vi "File Viewer v2.vi"() -> ()   [LabVIEW 2019]
uses:
  <vilib>/Utility/file.llb/Read Delimited Spreadsheet (I64).vi
panel:
  in  "Stop":bool
  in  "Tab Control":T1(tab)
  out "Raw Image From Camera":i32[][](graph)
  in  "file path for picture":path
  out "Expected position on spectrometer (pixels):":dbl
  in  "Grating:":u16(ring) items=["Shimadzu 30-006  "]
  in  "Laser:":u16(ring) items=["800nm  "]
  in  "Harmonic":dbl min=10.0 max=40.0
  out "l (nm)":dbl
  out "E (J)":dbl
  out "E (eV)":dbl
  out "Nearest Harmonic of 800nm":dbl
  out "Vertical Binned Waveform Graph":i64[](graph)
  out "Cursor Position (pixels)":dbl
  out "Distance to nearest harmonic of 800nm (pixels)":dbl
  in  "Caibration Date":u16(ring) items=["first calibration - 7/31", "7/31-current"]
  out "Wavelength Graph":cluster{"lamda (m)":dbl, "Numeric":i64}[](graph)
  out "Energy Graph (eV)":cluster{"lamda (m)":dbl, "Numeric":i64}[](graph)
  out "Harmonics Graph":cluster{"lamda (m)":dbl, "Numeric":i64}[](graph)
  in  "Pump/Probe Run Folder:":path
  out "XUV":dbl[][](graph)=[[0.0010313840536425023, 0.0010313840536425023, 0.0010274759814052766, 0.0010401531177745159, 0.00104452387932524, 0.0010522711712232782, 0.001047206375702307, 0.0010453914217880493, 0.0010393489196820073, 0.0010272942106035452, 0.0010408196107141979, 0.0010468510964080136, 0.001062026204249532, 0.001106433361933133, 0.001154520001300267, 0.0011934960677563772, 0.001214033414248973, 0.0012241024150236718, 0.0012391453259184763, 0.0012555680424446059, 0.0012925281054633312, 0.001352528994653044, 0.0014089853532089937, 0.0014660421062312687, 0.0015363130457188075, 0.0015691474623588406, 0.0016108363203256395, 0.0016140062929437132, 0.0015863330654316305, 0.001566139981821102, 0.0015480455247396548, 0.0015630250912641588, 0.0016089194645982896, 0.0016388896140595243, 0.0016752961023638853, 0.001688323009821305, 0.0016919033437948032, 0.0017147706614732288, 0.0017464097973867246, 0.001779717919752482, 0.001837171263614898, 0.00188523587015758, 0.001909243386501412, 0.0019293676175355272, 0.0019505631946586353, 0.0019533283141273984, 0.001977616748982997, 0.0019911972311547808, 0.002017708227177005, 0.002053718124641225, 0.0020883013967221585, 0.002112669700566397, 0.0021315656016372966, 0.0021208218456137463, 0.002105299720787104, 0.002099830072116822, 0.0021012126318512036, 0.0020908214010188896, 0.002095054457416787, 0.002100080695494967, 0.0021084586769929523, 0.0020993728910094368, 0.002104955457905037, 0.0020792872174181134, 0.0020928346503532183, 0.0020942117018814864, 0.002102964241395161, 0.0021093372358679877, 0.002121036665652156, 0.002136567052787968, 0.002154127213876447, 0.002169360157882152, 0.0021869395976920275, 0.0021825908689657556, 0.002171045668952753, 0.0021674267775364637, 0.0021489908116760054, 0.002157660728097984, 0.002145658346977596, 0.002135917084466625, 0.00209696855904108, 0.0020850653256307278, 0.0020535996982097935, 0.002049595232365589, 0.0020524236962046524, 0.0020767176392663643, 0.002111884781195284, 0.002137809153266466, 0.0021668842192343256, 0.00216397037820051, 0.0021656008072099796, 0.0021352698702483386, 0.0021013916485498785, 0.0020823029602650214, 0.0020479290000163844, 0.0020333460243320213, 0.0020002169186649392, 0.0019659586307446764, 0.0019358700548520106, 0.0019274369912928948, 0.0019173046461478957, 0.001900014387158957, 0.0018599917615413628, 0.001814549061108504, 0.0017608991335671654, 0.0017321325271416374, 0.0017011240808280886, 0.0016809695546603515, 0.0016804848325224012, 0.001677022924980334, 0.0016912533754734602, 0.0016999535870290603, 0.0017145172839920274, 0.001701024933118053, 0.0017087557003977521, 0.0017038864461937952, 0.0017154509249281934, 0.0017378638156022909, 0.001773105318313737, 0.0017971238510697952, 0.001824766783448256, 0.0018273914436611356, 0.0018233456662710829, 0.001811169776658133, 0.001808649772361402, 0.0017980740166243004, 0.0017838545825434003, 0.001763256645783561, 0.0017210445082360198, 0.001701132343137258, 0.0016754062664861471, 0.001664623953019805, 0.0016487024832499652, 0.0016273141189128994, 0.0016010950578146683, 0.0015728930425157306, 0.0015352912734848325, 0.0015149109108664593, 0.001483448037548582, 0.0014523514599372237, 0.0014315579818603703, 0.0014274984339550348, 0.0014181675327994876, 0.0014143999198181453, 0.0014053113797315735, 0.0013993515007172275, 0.001408693418285001, 0.0013985390403155494, 0.001397974449188959, 0.0013917694550025816, 0.0013787315311329358, 0.0013626448151797038, 0.0013449083914956062, 0.0013370509354753064, 0.001325880293477993, 0.0013185543793476045, 0.001294420174263172, 0.00127875483607759, 0.0012659041912157889, 0.0012433398248735822, 0.001228894554342046, 0.0012003400138518715, 0.001183988904005212, 0.0011747543964566436, 0.0011585547622780935, 0.0011605046672421217, 0.0011473565792502146, 0.0011370039058606926, 0.0011340652778993677, 0.0011226770617605876, 0.0011216442731143861, 0.0011107600578349525, 0.0011026409620242816, 0.0010866919512238764, 0.0010731362559796018, 0.001051089661012024, 0.0010301832647098524, 0.001009888279286232, 0.0009965887156262153, 0.0009909235256389188, 0.0009767536654130364, 0.0009747817276245561, 0.0009568910741692924, 0.000949947980363763, 0.000956703795161448, 0.0009593917997446279, 0.0009746082191319944, 0.0009815127554947322, 0.0009862085012061277, 0.0009848589907084247, 0.0009587748806599638, 0.0009397330121270677, 0.0009244532483694009, 0.0009160174307072283, 0.0009138141482619988, 0.0009141501488348964, 0.0009184162544694721, 0.0009130457535092251, 0.000912208506180038, 0.0009004897976744733, 0.0008954966088329721, 0.000888658170943591, 0.000878327530378521, 0.0008779392018475493, 0.0008724833236925496, 0.0008753007711193868, 0.0008733894235981503, 0.0008842763929806406, 0.0008803270091975667, 0.0008834474079606231, 0.0008812331091031674, 0.0008784927765619131, 0.0008838109495640858, 0.0008909550928927427, 0.000899184352825675, 0.0009081654828930417, 0.000914194214483801, 0.0009259542345352136, 0.0009387635678511666, 0.0009425339349355657, 0.0009425063939050002, 0.0009326494590656548, 0.0009267529244216092, 0.0009192645182108854, 0.0009126023429171226, 0.0009054058716303917, 0.0008956756255316468, 0.0008975015958581308, 0.0008902445343041561, 0.0008840973762819658, 0.0008824283898297043, 0.0008799772381093866, 0.000884678492026895, 0.0008933897199947213, 0.0008983829088362226, 0.000893860671617389, 0.0008973749071175302, 0.0009013435696219998, 0.0009055848883290665, 0.0009138995254567515, 0.0009202174378684471, 0.000930589389979365, 0.000922150818214136, 0.0009280666315795773, 0.0009267253833910438, 0.0009243623629685353, 0.0009317653919845064, 0.0009418922289233926, 0.0009494384712983037, 0.0009643051195974898, 0.0009718458537662879, 0.0009862966325039368, 0.0009917001827008621, 0.0009979795376697665, 0.001014038712592433, 0.0010172830459930335, 0.0010330585483008768, 0.0010469640146333317, 0.001060098332109956, 0.0010826544361429932, 0.0011030761103072145, 0.0011350760337211167, 0.0011531154087414334, 0.0011576624328877758, 0.0011768364983673857, 0.0011841624124977737, 0.0011999406689086737, 0.0012165093528967996, 0.0012281895039595726, 0.0012561601746017613, 0.0012707651831105765, 0.001307240523991351, 0.001333627585376031, 0.0013666217399933432, 0.0014024911782016796, 0.0014332324765187446, 0.0014678102403935655, 0.0014988241949132272, 0.0015329365153714935, 0.0015343879276822883, 0.0015720971067323913, 0.0016118636007657278, 0.001651087536496926, 0.0016970920739533186, 0.001745473402347502, 0.0017665615694514051, 0.0018051024876245825, 0.0018256783915599696, 0.0018815618966801597, 0.0018972630382054765, 0.0019475088943689358, 0.001967589059754146, 0.0019944801219981727, 0.0020293085092511383, 0.0020797967264835726, 0.002127649267090901, 0.002177592171918141, 0.002209096356781867, 0.0022576126362258207, 0.0022860239633570555, 0.002367479315357191, 0.00239798651491445, 0.002459918030346795, 0.002492961758819125, 0.0025305745442622493, 0.0025619850896220525, 0.0025918974029190997, 0.0026126908809959533, 0.0026649499864937407, 0.002671884817990101, 0.0027487573425041584, 0.0027664331759210126, 0.0028080311484869457, 0.002835572179052315, 0.002897776350687257, 0.0029281981730497637, 0.0029626547563900967, 0.002993387792397992, 0.0030170785868903222, 0.0030149964849795806, 0.0030319039236436605, 0.0030360240618162396, 0.0030334957952103388, 0.0030378693108641195, 0.003026379192912247, 0.0030242502712495446, 0.0030348563221202682, 0.0030418489897808152, 0.0030719182869520852, 0.0030982750532031434, 0.0030908086798168716, 0.0031010319103627363, 0.0031036813575031253, 0.0030762670156783568, 0.003066933360419753, 0.003042223547796504, 0.0030263378813663996, 0.003004663090311454, 0.0029920548065186284, 0.0029706664421815625, 0.0029578268137319874, 0.0029413352446294445, 0.0029132489016588815, 0.0028961762168114094, 0.002857943758180564, 0.00283680050901553, 0.0028030104186148787, 0.0027938640423641197, 0.0027516161014768444, 0.002719478472910115, 0.0026733913123620267, 0.002627637398283779, 0.0025728335015617514, 0.0025436510255746865, 0.002504355483164018, 0.0024615594757684913, 0.002436053727361903, 0.0024182842544411267, 0.0024007185851465346, 0.0023905779776923655, 0.0023550968680150007, 0.002333292634116398, 0.002292746728918062, 0.0022553735504408563, 0.0022384468330553806, 0.002203128215458351, 0.00217902430550754, 0.002143711196116624, 0.0021122262899742946, 0.0020506142504965077, 0.00203825383597877, 0.0020262487007553258, 0.0020074629638066875, 0.0019932738248594093, 0.0019544327094530695, 0.0019488088310116213, 0.0019049882972790627, 0.0018915620448784454, 0.0018528393559035367, 0.001821197465886984, 0.0017890212798774634, 0.0017354539754278208, 0.0016897689139259869, 0.001663423164087155, 0.0016456371665480398, 0.0016412085688331283, 0.001628644350689207, 0.0016130809143167168, 0.0016073331012377244, 0.001603339651805746, 0.0015941712427305346, 0.001588935692820058, 0.0015824029603699523, 0.00157714813173808, 0.0015643332902160138, 0.0015630746651191763, 0.0015527274999357675, 0.0015555421932595482, 0.0015637163711313498, 0.0015732180266764021, 0.001592557338339404, 0.001584653062567143, 0.0015960522951181493, 0.0016165015103129358, 0.0016268707083207973, 0.0016398039762742945, 0.001641899848700319, 0.0016484215647381982, 0.0016487190078683044, 0.0016555629539637985, 0.0016557612493838694, 0.0016741145921526312, 0.0017004658501975761, 0.0017330110860166727, 0.0017605190673453631, 0.0017664348807108045, 0.0017779084740443371, 0.001790398331405732, 0.0018131775177863488, 0.0018366452299310996, 0.0018605453362557267, 0.0018882543671075445, 0.0018984252696953353, 0.001914192509694009, 0.0019416316384462862, 0.0019781785860065308, 0.0020108477564631713, 0.0020298097560074277, 0.0020661143424986973, 0.002068810609391047, 0.002110609631480107, 0.002115869968318093, 0.0021256800834054774, 0.0021556667574850513, 0.002178443189762611, 0.0021840174943490416, 0.002213334921385877, 0.002212183706308245, 0.00223874152208243, 0.0022391546375409104, 0.002258397555596934, 0.0022739802706908193, 0.0023094503639559585, 0.002319709397841558, 0.002351866305129683, 0.002368812301236555, 0.0023749456887434623, 0.002389630566240917, 0.0023986777947816403, 0.00241149814450982, 0.0024190003212358263, 0.0024229882624616918, 0.002422095933071374, 0.002423731870286957, 0.0024201625527256847, 0.0024417767535133868, 0.0024415812121963724, 0.002455808908586442, 0.002457513698378438, 0.0024465385976981386, 0.0024522313287160006, 0.0024169705472831585, 0.0024148361174143426, 0.0023995701241719585, 0.0023793853028705996, 0.0023548297200185167, 0.002332361747283289, 0.0023205108418310103, 0.0022940521737668603, 0.0022523164960481005, 0.0022274744864781374, 0.0022039158889325208, 0.0021684926154193433, 0.0021411526343771015, 0.002118635087786856, 0.002083801192327777, 0.002047124801923875, 0.0020278653592495127, 0.0019697703093749233, 0.0019519264756716211, 0.0019212622922401392, 0.0018812286502103187, 0.0018427428140982722, 0.001812265909674635, 0.00175640994558501, 0.0017214080498394828, 0.0016736711815605288, 0.0016349457384825634, 0.0015946835058990505, 0.0015675610989982752, 0.0015259052902681545, 0.0014996366553149056, 0.001476708747369236, 0.001439175830914751, 0.0014011692087345419, 0.0013630882257718063, 0.0013162216540587178, 0.0012905451512626243, 0.0012539458757443056, 0.0012235736272368167, 0.0012001196856073486, 0.001185272316029558, 0.0011544346241055146, 0.0011379100057662933, 0.0010844501113358553, 0.0010647610285846733, 0.0010130802847287583, 0.0009929670701068693, 0.0009656849252288149, 0.0009476042386626501, 0.0009280005331062204, 0.0009123489654359212, 0.0008921173243826012, 0.0008740696870531149, 0.000861342976828858, 0.0008399518583887359, 0.0008269304591374295, 0.000805963472568014, 0.0007840931401960546, 0.0007730684656607372, 0.0007618757908389714, 0.000755502796366145, 0.0007484440302322409, 0.0007361304354664644, 0.0007236515945172958, 0.0007035631668229157, 0.0006909796699575985, 0.0006775396470416985, 0.0006603843391025302, 0.0006506954045496334, 0.0006404831904159946, 0.0006315406177914192, 0.000626814576946402, 0.0006201799426832045, 0.0006156053775062967, 0.0006078663479174281, 0.0005998298751984535, 0.0005900335306263518, 0.0005812644664943382, 0.0005748804556092857, 0.0005698349388097101, 0.000566761359798615, 0.0005616442363195694, 0.0005622749259195163, 0.0005532993040582626, 0.0005422911541412846, 0.0005348495676825219, 0.0005325361211150309, 0.0005320376284617976, 0.0005307018884793774, 0.0005264054877111798, 0.0005264054877111798, 0.0005228637111804734, 0.0005181238998201733, 0.0005176309153730532, 0.0005136154331166225, 0.0005124091359778592, 0.0005101562796776121, 0.0005055431570579128, 0.0004995529829099451, 0.0004920150028442035, 0.0004884759804165536, 0.00048560345092858563, 0.000481450263519328, 0.000479029406932632, 0.00047415189041950524, 0.00047243608421528277, 0.0004715299843096821, 0.00047353772543789753, 0.00047000971942247376, 0.0004698554896513077, 0.0004721276246729506, 0.0004682388311571205, 0.0004696351614067847, 0.0004644106279085342, 0.00046173088563452376, 0.0004594807834373332, 0.0004550053659704607, 0.0004509155229315034, 0.00044808430498938354, 0.0004430277717775818, 0.0004410696045043841, 0.00043787759906185783, 0.00043347929648056836, 0.0004299017166101269, 0.00042542354504019795, 0.00042215993291820175, 0.00041868425486085215, 0.000416883071461877, 0.0004110388647759057, 0.0004118981449295452, 0.00040788541677617095, 0.00040867033614728403, 0.00040761000647051725, 0.0004041866563712419, 0.00040178507850594175, 0.00039903372955246133, 0.0003977007436730975, 0.0003977310388067194, 0.00039884645054461687, 0.00039690480788975835, 0.000394671230310907, 0.0003933712936682215, 0.00039117076532604856, 0.0003899947633209073, 0.00038895095826247983, 0.00038990112381698505, 0.00038822662915861066, 0.0003852577060636639, 0.00038354740806555447, 0.0003831673418437523, 0.00038108523993301045, 0.00038199133983861106, 0.0003807712721845652, 0.0003789921216100424, 0.0003772350038599718, 0.00037759028315426514, 0.0003756155912627282, 0.0003736216206497954, 0.000373136898511845, 0.0003710079768491419, 0.0003707132878220925, 0.0003699917128212798, 0.00036924259678990177, 0.0003697686304737003, 0.000369484957858877, 0.0003692976788510325, 0.00037006056539769325, 0.00036974108944313496, 0.00036845492331573224, 0.0003671825277036122, 0.0003674441674939832, 0.00036729820003198675, 0.00036671708428705744, 0.0003670723635813507, 0.0003662516408705027, 0.0003653593114801848, 0.0003654336722627113, 0.00036621859163382426, 0.0003649076385789127, 0.0003645000313265452, 0.00036404009611610357, 0.00036481399907499045, 0.00036354435756592694, 0.0003624454704463687, 0.00036318632416857717, 0.000362616224835874, 0.00036201858447260554, 0.0003629026515537539, 0.00036316429134412485, 0.0003618092726403087, 0.00036178173160974337, 0.0003609059268377646, 0.0003606580575626763, 0.00035972441662651027, 0.00035978776099681063, 0.0003598290725426587, 0.0003593278257863689, 0.00035902487445014993, 0.0003587962838964574, 0.00035836939792269413, 0.00035583837721373673, 0.0003554059830338604, 0.0003547532606094612, 0.0003549102444836838, 0.00035429057129596295, 0.0003543126041204152, 0.0003549185067928534, 0.0003548248672889311, 0.00035513057272820676, 0.0003544998831282598, 0.00035434014515098067, 0.000354516407746599, 0.00035333489753534467, 0.0003535855209134895, 0.0003530154215807864, 0.0003527152243476239, 0.0003532798154742139, 0.00035263260125592777, 0.0003519964034498677, 0.000351608074918896, 0.00035093882787615757, 0.000349443349916458, 0.00034942957940117537, 0.0003491624314046913, 0.00034956453045094566, 0.00034901095573658175, 0.00034910184113744744, 0.0003489310867479422, 0.0003488181685226241, 0.0003479836752964935, 0.0003476917403725006, 0.00034843259409470895, 0.0003489586277785075, 0.0003480910853156984, 0.0003474548875096384, 0.0003469619030625183, 0.00034665344352018617, 0.0003463918037298151, 0.00034654052529486815, 0.00034605304905386115, 0.0003454196053508576, 0.00034516347376659963, 0.00034559862204953256, 0.0003448357355028718, 0.0003449403914190202, 0.00034430419361296017, 0.00034424635744877293, 0.000344852260121211, 0.0003448384896059283, 0.0003451028834993559, 0.0003437423565894266, 0.0003425580922751158, 0.00034259664971790727, 0.0003416354677511759, 0.00034174838597649394, 0.00034173461546121124, 0.0003417869434192854, 0.0003409965158420593, 0.00034094143378092864, 0.0003408477942770064, 0.0003402501539137379, 0.0003404980231888262, 0.0003398783500011054, 0.00033904936498108774, 0.00033842969179336696, 0.00033828372433137053, 0.0003380661501899041, 0.00033740791955939176, 0.000338358085113897, 0.0003377081167925543, 0.00033727847671573453, 0.000337388640837996, 0.00033701959102842003, 0.00033749605085720095, 0.00033774116602923275, 0.0003364384752834908, 0.000335931720321088, 0.0003357031297673954, 0.00033592070390886183, 0.0003353395881639325, 0.00033492922680850853, 0.00033513303043469225, 0.00033468961984258985, 0.0003348713906443213, 0.00033494024322073466, 0.0003348108003770775, 0.00033487689885043436, 0.00033441145543387964, 0.0003341993894985263, 0.0003345464064836499, 0.00033424896335354395, 0.00033390194636842026, 0.00033334837165405635, 0.00033337040447850867, 0.0003331583385431553, 0.0003329132233711235, 0.0003332326993256818, 0.0003335301424557878, 0.0003335026014252224, 0.00033401761869679484, 0.0003333428634479433, 0.00033282509207331433, 0.00033313630571870306, 0.0003330839777606288, 0.00033270666564188324, 0.00033214758272140626, 0.00033204843501137094, 0.00033124974512497527, 0.0003311781384455053, 0.00033189695934326144, 0.0003313213518044452, 0.0003320980088663886, 0.0003318336149729611, 0.00033207873014499283, 0.0003325304030462649, 0.0003314094831022544, 0.00033175650008737803]]
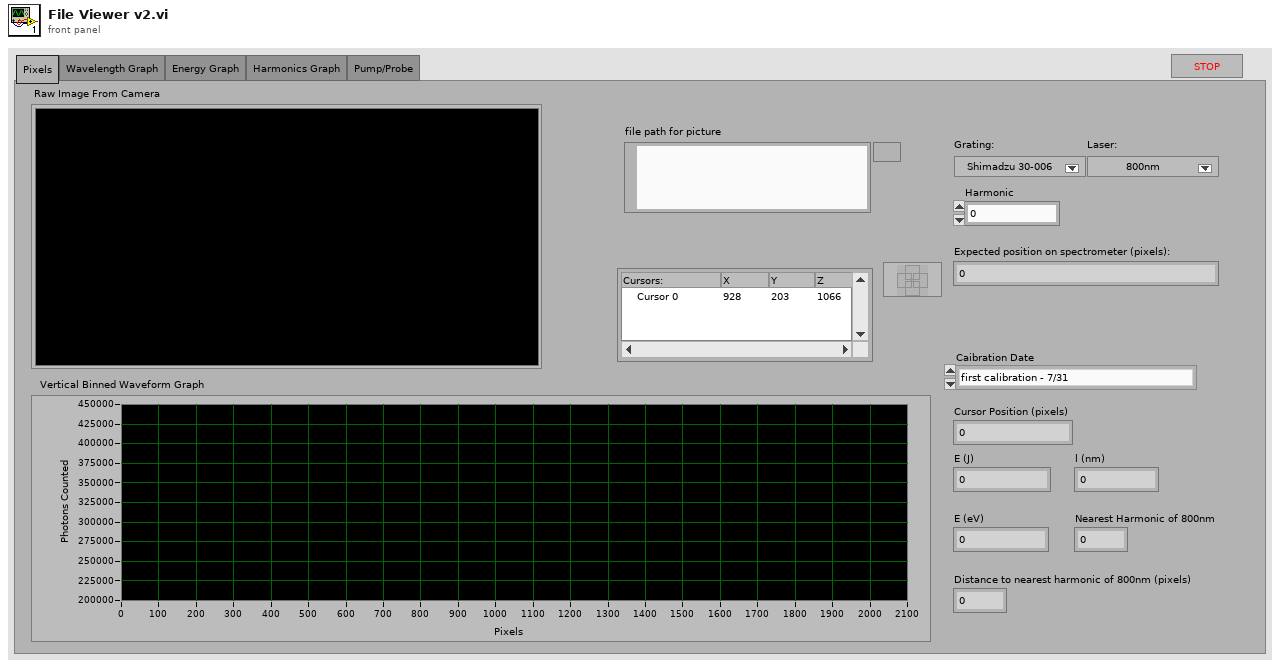
[diagram p1: front panel]
types:
  T1 = enum32{"Pixels", "Wavelength Graph", "Energy Graph", "Harmonics Graph", "Pump/Probe"}
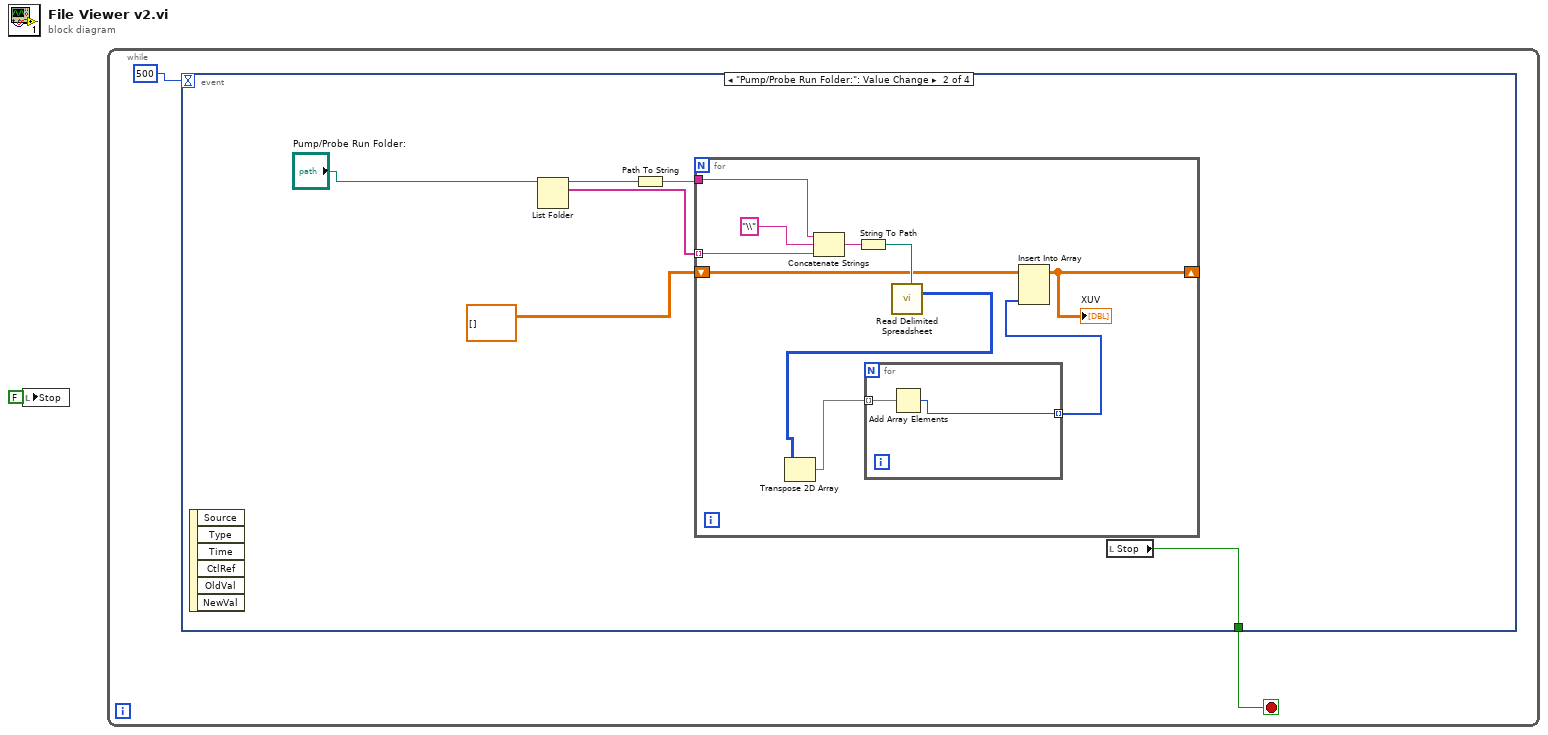
[diagram p0: block diagram]
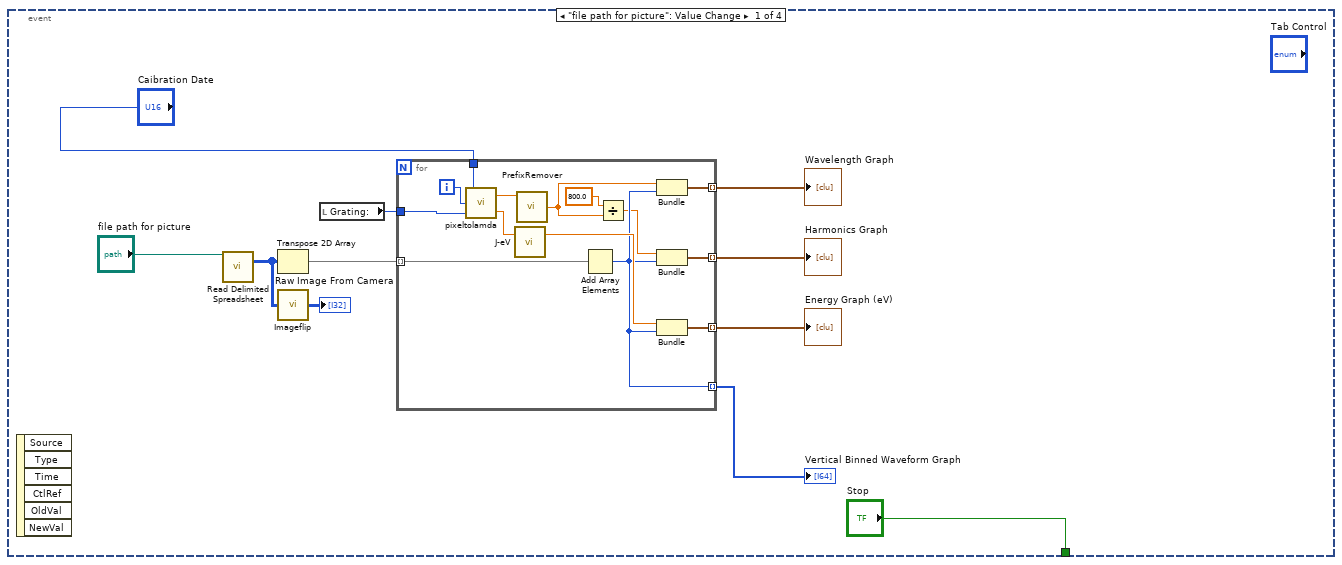
[diagram p2: hidden frame]
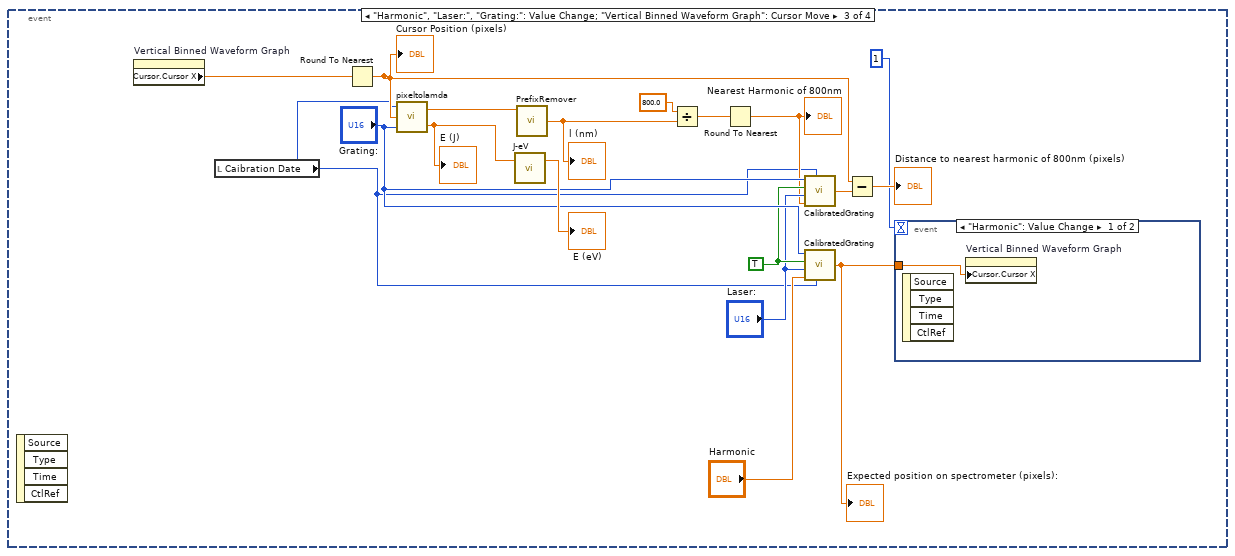
[diagram p3: hidden frame]
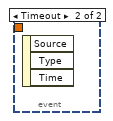
[diagram p4: hidden frame]
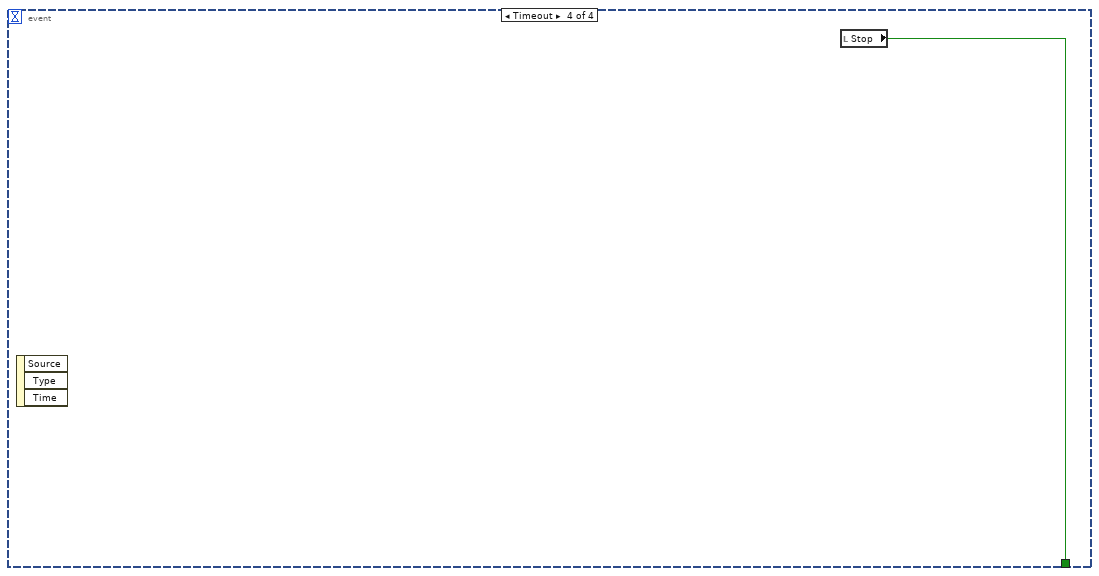
[diagram p5: hidden frame]
diagram:
  n1 = local write "Stop"(FALSE) -> ()
  n2 = while {
    stop <- w3 stop-if-true
    n3 = event shown="[1] \"Pump/Probe Run Folder:\": Value Change" {
      selector: _ -> [_ _ _ _]
      dyn-events: _ -> [_ _ _ _]
      timeout: 500 -> [_ _ _ _]
      tunnel: ["Stop" w30 _ w66] -> w3
      event "file path for picture": Value Change {
        n4 = event-data() -> ()  [unwired: 1 in, 6 out]
        n5 = call-poly <vilib>:"Read Delimited Spreadsheet.vi"("file path (dialog if empty)"="file path for picture") -> ("all rows"=w11:i64[][])  [unwired: 9 in, 5 out]
        n6 = Transpose 2D Array(2D array=w11) -> (transposed array=w10:i64[][])
        n7 = call "Imageflip.vi"("2D array"=w11) -> ("transposed array"=→"Raw Image From Camera":i32[][])
        n8 = local read "Grating:"() -> (w8:u16)
        n9 = for {
          tunnel: w10 -> [w28] mode=indexing
          tunnel: [w21] -> w9 mode=indexing
          tunnel: w8 -> [w26]
          tunnel: [w25] -> w7 mode=indexing
          tunnel: [w22] -> w6 mode=indexing
          tunnel: [w16] -> w5 mode=indexing
          tunnel: "Caibration Date" -> [w15]
          i -> [w27]
          n10 = call "pixeltolamda.vi"("Grating:"=w26, "Pixel Postion"=w27, "Caibration Date"=w15) -> ("E (J)"=w24:dbl, "lamda (m)"=w19:dbl)
          n11 = call "J-eV.vi"("J"=w24) -> ("eV"=w23:dbl)  [unwired: 1 in, 1 out]
          n12 = call "PrefixRemover.vi"("Nano"=w19) -> ("No prefix"=w18:dbl)  [unwired: 3 in]
          n13 = Add Array Elements(numeric array=w28) -> (sum=w21:i64)
          n14 = Divide(x=800.0, y=w18) -> (x/y=w17:dbl)
          n15 = Bundle("No prefix"=w18, "Numeric"=w21) -> (w25:cluster{"No prefix":dbl, "Numeric":i64})  [unwired: 1 in]
          n16 = Bundle(w17, "Numeric"=w21) -> (w16:cluster{dbl, "Numeric":i64})  [unwired: 1 in]
          n17 = Bundle("eV"=w23, "Numeric"=w21) -> (w22:cluster{"eV":dbl, "Numeric":i64})  [unwired: 1 in]
        }
        "Vertical Binned Waveform Graph" <- w9
        "Wavelength Graph" <- w7
        "Energy Graph (eV)" <- w6
        "Harmonics Graph" <- w5
      }
      event "Pump/Probe Run Folder:": Value Change {
        n18 = event-data() -> ()  [unwired: 1 in, 6 out]
        n19 = List Folder(path="Pump/Probe Run Folder:") -> (path out=w32:path, filenames=w33:string[])  [unwired: 3 in, 2 out]
        n20 = Path To String(path=w32) -> (string=w31:string)
        n21 = for {
          tunnel: w33 -> [w42] mode=indexing
          tunnel: w31 -> [w40]
          shift-right: [w35] -> _
          shift-left: dbl[][] [] -> [w39]
          n22 = Concatenate Strings(w40, "\\" ("string"), w42) -> (w44:string)
          n23 = String To Path(string=w44) -> (path=w43:path)
          n24 = call-poly <vilib>:"Read Delimited Spreadsheet.vi"("file path (dialog if empty)"=w43) -> ("all rows"=w37:i64[][])  [unwired: 9 in, 5 out]
          n25 = Transpose 2D Array(2D array=w37) -> (transposed array=w36:i64[][])
          n26 = for {
            tunnel: w36 -> [w46] mode=indexing
            tunnel: [w45] -> w38 mode=indexing
            n27 = Add Array Elements(numeric array=w46) -> (sum=w45:i64)
          }
          n28 = Insert Into Array(array=w39, new element=w38) -> (w35:dbl[][])  [unwired: 2 in]
          "XUV" <- w35
        }
        n29 = local read "Stop"() -> (w30:bool)
      }
      event "Harmonic", "Laser:", "Grating:": Value Change; "Vertical Binned Waveform Graph": Cursor Move {
        w56 = TRUE ("Subvi?")
        n30 = event-data() -> ()  [unwired: 1 in, 4 out]
        n31 = property on="Vertical Binned Waveform Graph" class="WFGraph (strict)"() -> ("Cursor.Cursor X"=w58:dbl)  [unwired: 2 in, 2 out]
        n32 = local read "Caibration Date"() -> (w47:u16)
        n33 = Round To Nearest(number=w58) -> (nearest integer value=w50:dbl)
        "Cursor Position (pixels)" <- w50
        n34 = call "pixeltolamda.vi"("Grating:"="Grating:", "Pixel Postion"=w50, "Caibration Date"=w47) -> ("E (J)"=w62:dbl, "lamda (m)"=w63:dbl)
        "E (J)" <- w62
        n35 = call "J-eV.vi"("J"=w62) -> ("eV"=→"E (eV)":dbl)  [unwired: 1 in, 1 out]
        n36 = call "PrefixRemover.vi"("Nano"=w63) -> ("No prefix"=w53:dbl)  [unwired: 3 in]
        "l (nm)" <- w53
        n37 = Divide(x=800.0, y=w53) -> (x/y=w60:dbl)
        n38 = Round To Nearest(number=w60) -> (nearest integer value=w54:dbl)
        "Nearest Harmonic of 800nm" <- w54
        n39 = call "CalibratedGrating.vi"("Grating:"="Grating:", "Subvi?"=w56, "Laser:"="Laser:", "Harmonic"=w54, "Caibration Date"=w47) -> ("Position on spectrometer (pixels):"=w52:dbl)
        n40 = call "CalibratedGrating.vi"("Grating:"="Grating:", "Subvi?"=w56, "Laser:"="Laser:", "Harmonic"="Harmonic", "Caibration Date"=w47) -> ("Position on spectrometer (pixels):"=w49:dbl)
        "Expected position on spectrometer (pixels):" <- w49
        n41 = Subtract(x=w50, y=w52) -> (x-y=→"Distance to nearest harmonic of 800nm (pixels)":dbl)
        n42 = event shown="[0] \"Harmonic\": Value Change" {
          selector: _ -> [_ _]
          dyn-events: _ -> [_ _]
          timeout: 1 -> [_ _]
          tunnel: w49 -> [w65 _]
          event "Harmonic": Value Change {
            n43 = event-data() -> ()  [unwired: 1 in, 4 out]
            n44 = property on="Vertical Binned Waveform Graph" class="WFGraph (strict)"("Cursor.Cursor X"=w65) -> ()  [unwired: 2 in, 2 out]
          }
          event Timeout {
            n45 = event-data() -> ()  [unwired: 1 in, 3 out]
          }
        }
      }
      event Timeout {
        n46 = event-data() -> ()  [unwired: 1 in, 3 out]
        n47 = local read "Stop"() -> (w66:bool)
      }
    }
  }
